vi "Create.vi"(8 "error in (no error)":errorcluster caption="错误输入（无错误）", 9 "Length":i32=256, 10 "Color Segement":u32[](array[colorbox])=[16448250, 0, 16736786, 1198079], 11 "Scroll Gradient 输入":refnum<class "Scroll Gradient.lvclass"> caption="DNL_LabVIEW Object in") -> (0 "error out":errorcluster caption="错误输出", 3 "Scroll Gradient 输出":refnum<class "Scroll Gradient.lvclass"> caption="DNL_LabVIEW Object out")   [LabVIEW 2011, in "Scroll Gradient.lvclass"]
uses:
  Scroll Gradient.lvclass
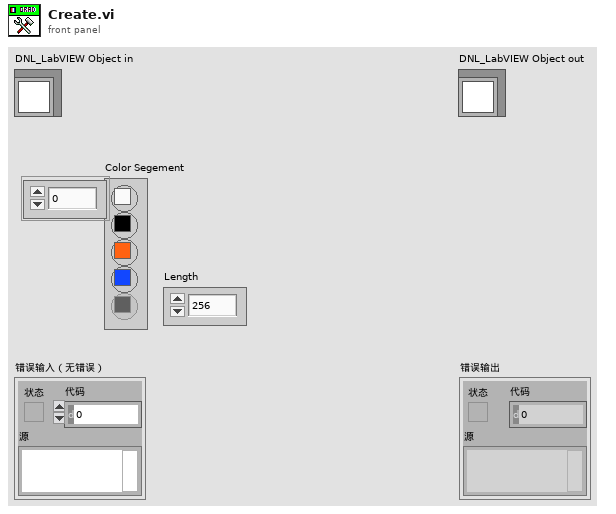
[diagram p1: front panel]
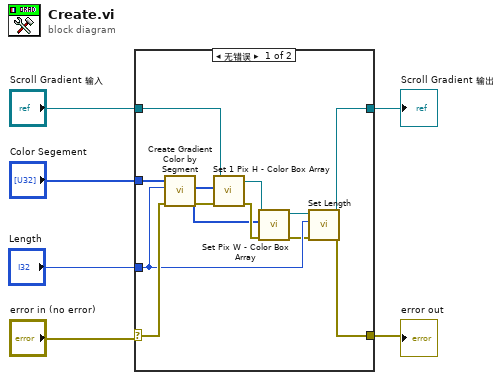
[diagram p0: block diagram]
diagram:
  n1 = case shown="无错误" "error in (no error)" {
    selector: "error in (no error)" -> [w18 w21]
    tunnel: [w7 w21] -> w5
    tunnel: [w8 w20] -> w3
    tunnel: "Scroll Gradient 输入" -> [w17 w20]
    tunnel: "Color Segement" -> [w19 _]
    tunnel: "Length" -> [w11 _]
    frame No Error {
      n2 = call "Create Gradient Color by Segment.vi"("错误输入"=w18, "Length"=w11, "Color Segement"=w19) -> ("错误输出"=w15:errorcluster, "1 Pix W - Color Box Array"=w12:u32[], "1 Pix H - Color Box Array"=w16:u32[])  [unwired: 6 in]
      n3 = call "Set 1 Pix H - Color Box Array.vi"("error in (no error)"=w15, "1 Pix H - Color Box Array"=w16, "Scroll Gradient输入"=w17) -> ("error out"=w13:errorcluster, "Scroll Gradient输出"=w14:refnum<class "Scroll Gradient.lvclass">)  [unwired: 7 in]
      n4 = call "Set Pix W - Color Box Array.vi"("error in (no error)"=w13, "1 Pix W - Color Box Array"=w12, "Scroll Gradient输入"=w14) -> ("error out"=w9:errorcluster, "Scroll Gradient输出"=w10:refnum<class "Scroll Gradient.lvclass">)  [unwired: 7 in]
      n5 = call "Set Length.vi"("error in (no error)"=w9, "Length"=w11, "Scroll Gradient输入"=w10) -> ("error out"=w7:errorcluster, "Scroll Gradient输出"=w8:refnum<class "Scroll Gradient.lvclass">)  [unwired: 7 in]
    }
    frame Error {
    }
  }
  "error out" <- w5
  "Scroll Gradient 输出" <- w3
